vi "findNextAvailableDriveLetter.vi"(8 "error in (no error)":errorcluster) -> (0 "error out":errorcluster, 3 "Next Available Disk Letter":string)   [LabVIEW 2017, in "BuildWorker Controller.lvlib" / "BuildWorker Controller.lvclass"]
uses:
  BuildWorker Controller.lvclass
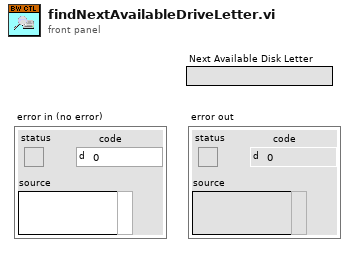
[diagram p1: front panel]
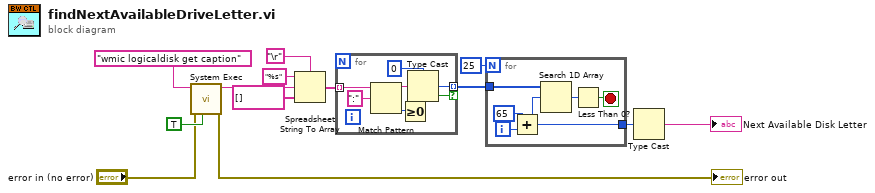
[diagram p0: block diagram]
diagram:
  n1 = call <vilib>:"System Exec.vi"("run minimized? (F)"=TRUE, "error in (no error)"="error in (no error)", "command line"="wmic logicaldisk get caption") -> ("error out"=→"error out":errorcluster, "standard output"=w8:string)  [unwired: 5 in, 2 out]
  n2 = Spreadsheet String To Array(delimiter (Tab)="\r", format string="%s", spreadsheet string=w8, array type (2D Dbl)=string[] []) -> (array=w7:string[])
  n3 = for {
    tunnel: w7 -> [w20] mode=indexing
    tunnel: [w15] -> w6 mode=indexing if=w17
    n4 = Match Pattern(string=w20, regular expression=":") -> (before substring=w16:string, offset past match=w18:i32)  [unwired: 1 in, 2 out]
    n5 = Greater Or Equal To 0?(x=w18) -> (x >= 0?=w17:bool)
    n6 = Type Cast(type=u8 0, x=w16) -> (*(type *) &x=w15:u8)
  }
  n7 = for {
    N: 25 -> [_]
    tunnel: w6 -> [w26]
    tunnel: [w21] -> w4
    i -> [w25]
    stop <- w22 stop-if-true
    n8 = Add(x=65, y=w25) -> (x+y=w21:i32)
    n9 = Search 1D Array(1D array=w26, element=w21) -> (index of element=w23:i32)  [unwired: 1 in]
    n10 = Less Than 0?(x=w23) -> (x < 0?=w22:bool)
  }
  n11 = Type Cast(x=w4) -> (*(type *) &x=→"Next Available Disk Letter":string)  [unwired: 1 in]
